vi "SavePattern.vi"(8 "Error In":errorcluster, 10 "Pattern":T1, 11 "Pattern Save Path":path) -> (0 "Error Out":errorcluster, 3 "XML":string)   [LabVIEW 2012, in "Virtual-PGA.lvlib"]
doc: "This VI saves a pattern to a XML file. The \"Select Pattern Save File Path\" VI should be used to select the file."
uses:
  Virtual-PGA.lvlib
  Controls/Pattern.ctl
  Controls/Input.ctl
  <vilib>/xml/Close Reference(Node).vi
  <resource>/objmgr/DOMUserDefRef.rc
  <vilib>/xml/NI_XML.lvlib
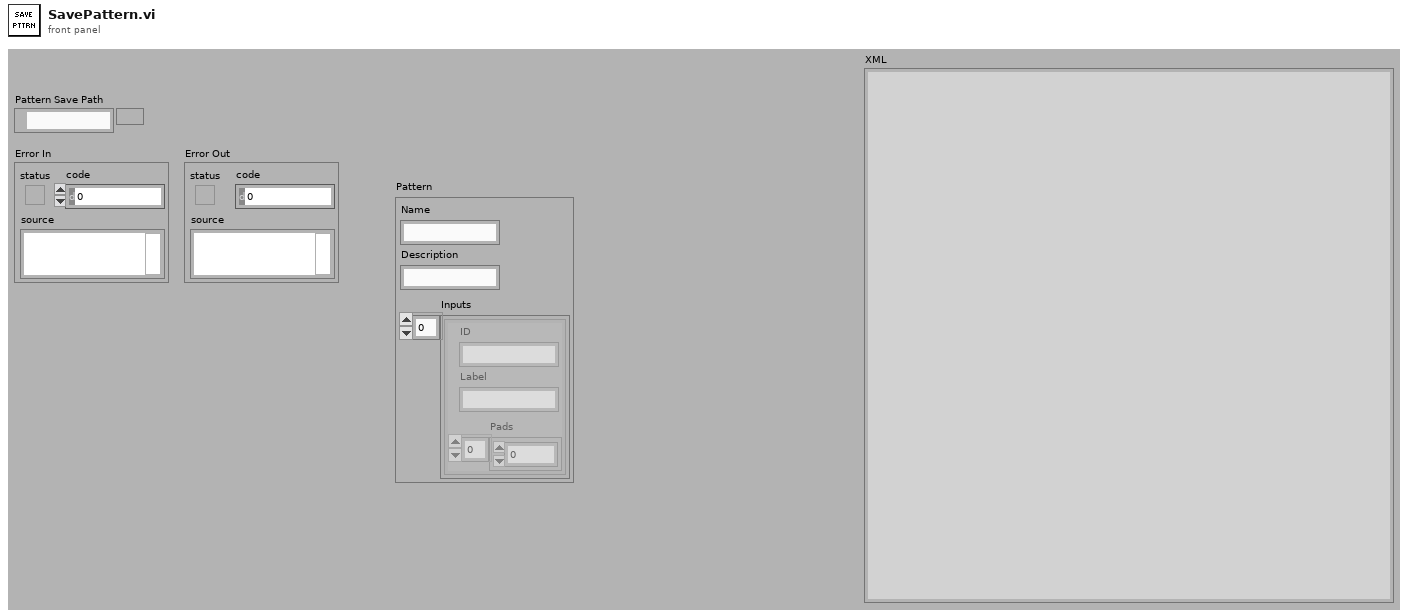
[diagram p1: front panel]
types:
  T1 = typedef "Virtual-PGA.lvlib/Pattern.ctl" = cluster{"Name":string, "Description":string, "Inputs":T2[]}
  T2 = typedef "Virtual-PGA.lvlib/Input.ctl" = cluster{"ID":string, "Label":string, "Pads":u32[]}
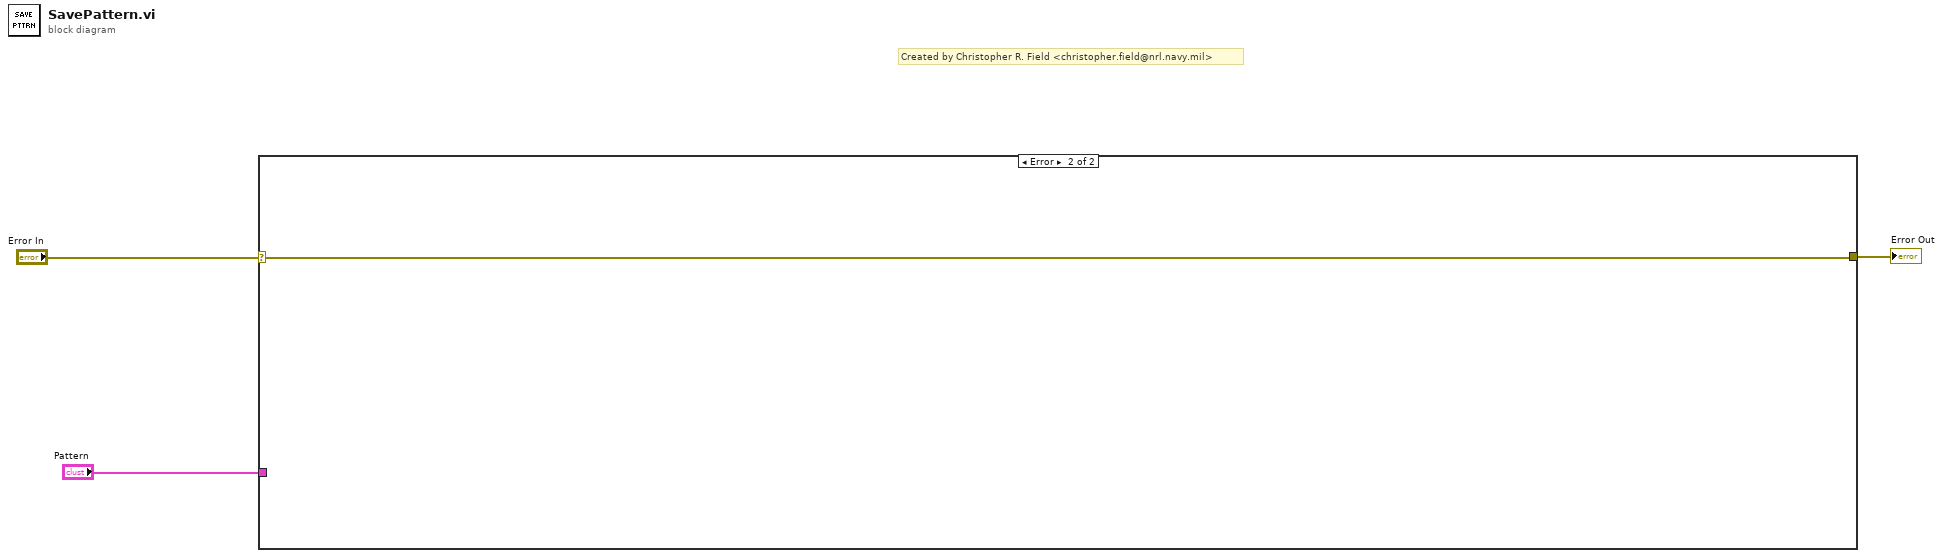
[diagram p0: block diagram]
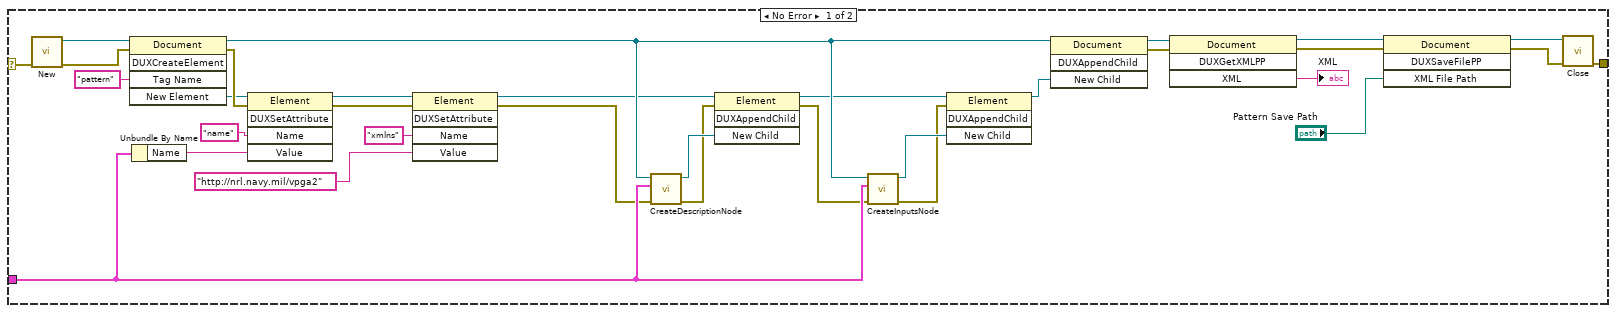
[diagram p2: hidden frame]
diagram:
  # "Created by Christopher R. Field <christopher.field@nrl.navy.mil>"
  n1 = case shown="Error" "Error In" {
    selector: "Error In" -> [w4 w35]
    tunnel: [w20 w35] -> w3
    tunnel: "Pattern" -> [w15 _]
    frame No Error {
      n2 = call <vilib>:"New.vi"("error in (no error)"=w4) -> ("error out"=w32:errorcluster, "DOM document out"=w14:refnum<k20>)  [unwired: 7 in]
      n3 = invoke class="Document" method="DUXCreateElement"(reference=w14, error in=w32, "Tag Name"="pattern") -> (error out=w31:errorcluster, "New Element"=w13:refnum<k20>)  [unwired: 2 in, 3 out]
      n4 = Unbundle By Name(w15) -> ("Name"=w16:string)
      n5 = invoke class="Element" method="DUXSetAttribute"(reference=w13, error in=w31, "Name"="name", "Value"=w16) -> (reference out=w12:refnum<k20>, error out=w11:errorcluster)  [unwired: 1 in, 3 out]
      n6 = invoke class="Element" method="DUXSetAttribute"(reference=w12, error in=w11, "Name"="xmlns", "Value"="http://nrl.navy.mil/vpga2") -> (reference out=w9:refnum<k20>, error out=w10:errorcluster)  [unwired: 1 in, 3 out]
      n7 = call "CreateDescriptionNode.vi"("Error In"=w10, "Pattern"=w15, "DOM Document"=w14) -> ("Error out"=w29:errorcluster, "Description Node"=w30:refnum<k20>)  [unwired: 7 in]
      n8 = invoke class="Element" method="DUXAppendChild"(reference=w9, error in=w29, "New Child"=w30) -> (reference out=w6:refnum<k20>, error out=w5:errorcluster)  [unwired: 1 in, 2 out]
      n9 = call "CreateInputsNode.vi"("Error In"=w5, "Pattern"=w15, "DOM Document"=w14) -> ("Error out"=w27:errorcluster, "Inputs Node"=w28:refnum<k20>)  [unwired: 7 in]
      n10 = invoke class="Element" method="DUXAppendChild"(reference=w6, error in=w27, "New Child"=w28) -> (reference out=w19:refnum<k20>)  [unwired: 1 in, 3 out]
      n11 = invoke class="Document" method="DUXAppendChild"(reference=w14, "New Child"=w19) -> (reference out=w18:refnum<k20>, error out=w17:errorcluster)  [unwired: 2 in, 2 out]
      n12 = invoke class="Document" method="DUXGetXMLPP"(reference=w18, error in=w17) -> (reference out=w25:refnum<k20>, error out=w24:errorcluster, "XML"=→"XML":string)  [unwired: 2 in, 1 out]
      n13 = invoke class="Document" method="DUXSaveFilePP"(reference=w25, error in=w24, "XML File Path"="Pattern Save Path") -> (reference out=w22:refnum<k20>, error out=w21:errorcluster)  [unwired: 1 in, 2 out]
      n14 = call-poly <vilib>:"Close.vi"("error in (no error)"=w21, "node"=w22) -> ("error out"=w20:errorcluster)  [unwired: 7 in]
    }
    frame Error {
    }
  }
  "Error Out" <- w3
